vi "145-optim.vi"() -> ()   [LabVIEW 2021]
panel:
  out "size(s)":u64
  in  "Limit":i32
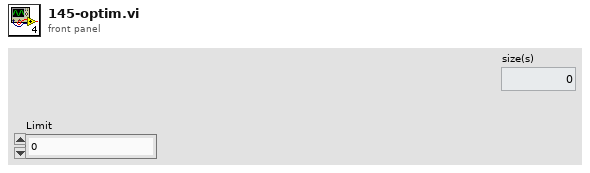
[diagram p1: front panel]
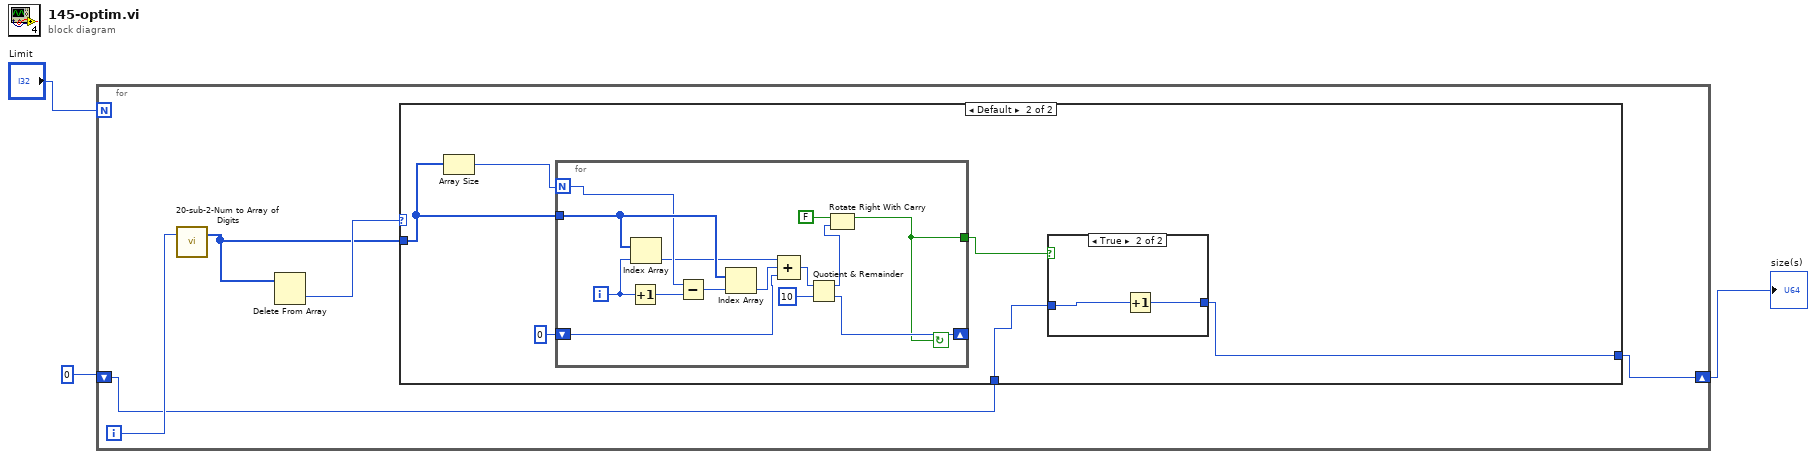
[diagram p0: block diagram]
diagram:
  n1 = for {
    N: "Limit" -> [_]
    shift-right: [w4] -> w1
    shift-left: u64 0 -> [w5]
    i -> [w8]
    n2 = call "20-sub-2-Num to Array of Digits.vi"("N"=w8) -> ("N as Array"=w6:u8[])  [unwired: 2 in]
    n3 = Delete From Array(array=w6) -> (deleted portion=w7:u8)  [unwired: 2 in, 1 out]
    n4 = case shown="Default" w7 {
      tunnel: w6 -> [_ w14]
      tunnel: w5 -> [w9 w11]
      tunnel: [w9 w10] -> w4
      frame 0 {
        # "Ends in zero. So reverse will have leading zero"
      }
      frame Default {
        n5 = Array Size(array=w14) -> (size(s)=w15:i32)
        n6 = for {
          N: w15 -> [w30]
          tunnel: w14 -> [w32]
          shift-right: [w22] -> _
          shift-left: u8 0 -> [w25]
          tunnel: [w19] -> w12
          i -> [w29]
          stop <- w19 continue-if-true
          n7 = Increment(x=w29) -> (x+1=w28:i32)
          n8 = Index Array(array=w32, index=w29) -> (element=w27:u8)
          n9 = Subtract(x=w30, y=w28) -> (x-y=w31:i32)
          n10 = Index Array(array=w32, index=w31) -> (element=w26:u8)
          n11 = Compound Arithmetic op=ADD(w27, w26, w25) -> (w24:u8)
          n12 = Quotient & Remainder(x=w24, y=u8 10) -> (x-y*floor(x/y)=w21:u8, floor(x/y)=w22:u8)
          n13 = Rotate Right With Carry(2:w21, 3:FALSE ("carry")) -> (1:w19:bool)  [unwired: 1 out]
        }
        n14 = case shown="True" w12 {
          tunnel: [w16 w17] -> w10
          tunnel: w11 -> [w16 w18]
          frame False {
          }
          frame True {
            n15 = Increment(x=w18) -> (x+1=w17:u64)
          }
        }
      }
    }
  }
  "size(s)" <- w1
